vi "Do Request.vi"(7 "Processing In":refnum<class "Processing.lvclass">, 11 "ConfigHTTPController in":refnum<class "ConfigHTTPController.lvclass">) -> (0 "error out":errorcluster, 5 "Processing":refnum<class "Processing.lvclass">)   [LabVIEW 2023, in "Volatus.lvlib" / "ConfigHTTPController.lvclass"]
doc: "A controller's main job is to respond to a request by generating a response. The response value must be specified by calling Set Response.vi on the Processing class that's passed through the VI otherwise an error will be generated.\n\nThere are several helpers available for common response types:\nGenerating HTML content programmatically - Create Basic Response.vi\nStreaming a file from disk - Create File Response.vi\nRedirecting the user to another URL - Create Redirect Response.vi\n\nFile responses are streamed in chunks and do not load the entire file into memory at once to send in the response which allows serving large files more efficiently."
uses:
  ConfigHTTPController.lvclass
  lv-http-server/HTTP Server/Processing/Processing.lvclass
  lv-http-server/HTTP Server/Processing/Processing.lvclass/Processing.ctl
  lv-http-util/HTTP Utils/Request/Request.lvclass/Request.ctl
  lv-uri/URI/URI/URI.lvclass/URI.ctl
  ConfigInfoValue/ConfigInfoValue.lvclass
  ConfigHTTPController.lvclass/ConfigHTTPController.ctl
  MessageQ/MessageQ.lvclass/MessageQ.ctl
  lv-http-util/HTTP Utils/Request/Get Target URI.vi
  lv-uri/URI/URI/Path String.vi
  lv-http-util/HTTP Utils/File Response/File Response.lvclass
  MessageQ/MessageQ.lvclass
  lv-http-util/HTTP Utils/Response/Response.lvclass
  lv-http-util/HTTP Utils/Request/Request.lvclass
  lv-http-util/HTTP Utils/FormField/FormField.lvclass
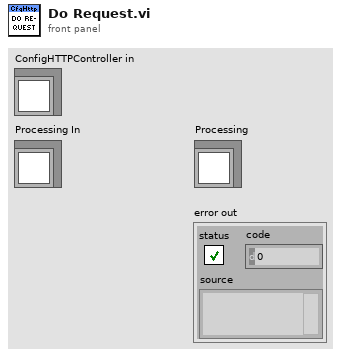
[diagram p1: front panel]
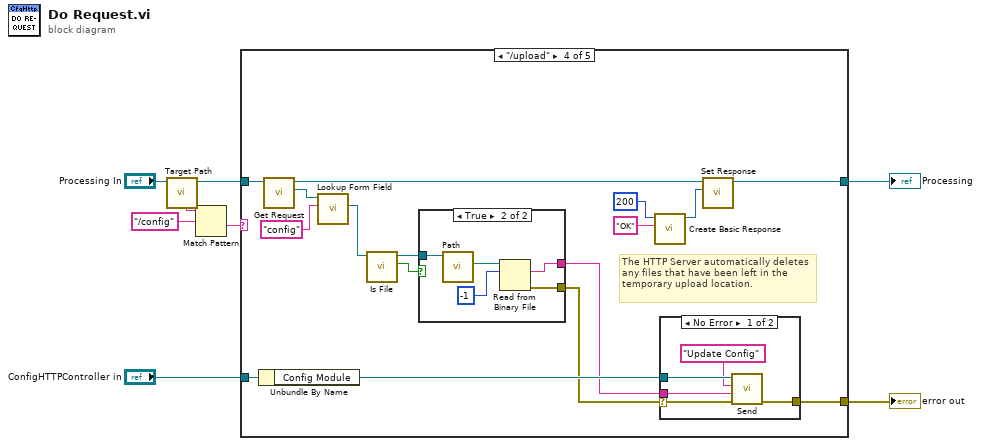
[diagram p0: block diagram]
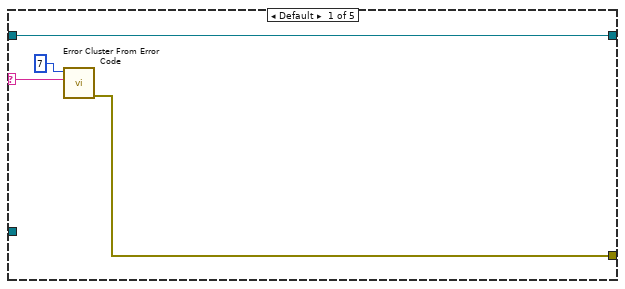
[diagram p2: hidden frame]
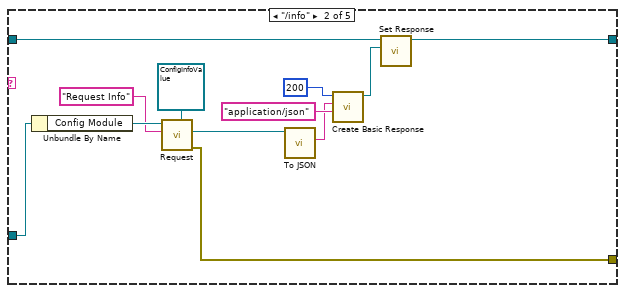
[diagram p3: hidden frame]
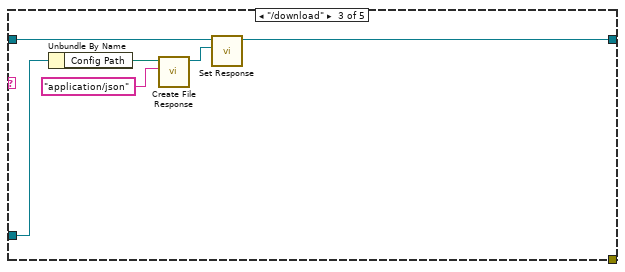
[diagram p4: hidden frame]
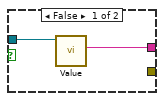
[diagram p6: hidden frame]
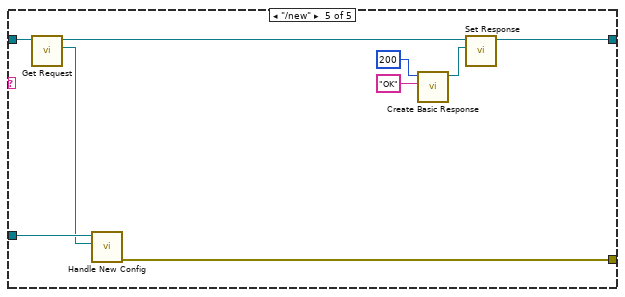
[diagram p7: hidden frame]
diagram:
  n1 = call "Target Path.vi"("Processing in"="Processing In") -> ("Processing out"=w3:refnum<class "Processing.lvclass">, "Target Path"=w7:string)  [unwired: 9 in]
  n2 = Match Pattern(string=w7, regular expression="/config") -> (after substring=w5:string)  [unwired: 1 in, 3 out]
  n3 = case shown="\"/upload\"" w5 {
    selector: w5 -> [w12 _ _ _ _]
    tunnel: [w10 w13 _ w41 w66] -> w4
    tunnel: w3 -> [w9 w16 w27 w46 w68]
    tunnel: "ConfigHTTPController in" -> [_ w24 w30 w43 w67]
    tunnel: [w9 w14 w25 w32 w60] -> w1
    frame Default {
      n4 = call <vilib>:"Error Cluster From Error Code.vi"("error message (\"\")"=w12, "error code (0)"=7) -> ("error out"=w10:errorcluster)  [unwired: 7 in]
    }
    frame "/info" {
      n5 = Unbundle By Name(w24) -> ("Config Module"=w23:refnum<class "MessageQ.lvclass">)
      n6 = call "Request.vi"("Response Type (None)"=refnum<class "ConfigInfoValue.lvclass"> refnum ("Volatus:ConfigInfoValue.lvclass"), "ID"="Request Info", "MessageQ in"=w23) -> ("error out"=w13:errorcluster, "Response"=w20:refnum<class "ConfigInfoValue.lvclass">)  [unwired: 6 in, 1 out]
      n7 = call "To JSON.vi"("ConfigInfoValue in"=w20) -> ("JSON string"=w17:string)  [unwired: 10 in]
      n8 = call "Create Basic Response.vi"("Content-Type (text/plain)"="application/json", "Payload"=w17, "Status Code"=u16 200) -> ("Response out"=w15:refnum<class "Response.lvclass">)  [unwired: 7 in, 1 out]
      n9 = call "Set Response.vi"("Response"=w15, "Processing in"=w16) -> ("Processing out"=w14:refnum<class "Processing.lvclass">)  [unwired: 9 in]
    }
    frame "/download" {
      n10 = Unbundle By Name(w30) -> ("Config Path"=w29:path)
      n11 = call "Create File Response.vi"("Content-Type (Auto)"="application/json", "Path"=w29) -> ("File Response out"=w26:refnum<class "File Response.lvclass">)  [unwired: 8 in, 1 out]
      n12 = call "Set Response.vi"("Response"=w26, "Processing in"=w27) -> ("Processing out"=w25:refnum<class "Processing.lvclass">)  [unwired: 9 in]
    }
    frame "/upload" {
      # "The HTTP Server automatically deletes any files that have been left in the temporary upload location."
      n13 = Unbundle By Name(w43) -> ("Config Module"=w42:refnum<class "MessageQ.lvclass">)
      n14 = call "Get Request.vi"("Processing in"=w46) -> ("Request"=w45:refnum<class "Request.lvclass">, "Processing out"=w44:refnum<class "Processing.lvclass">)  [unwired: 9 in]
      n15 = call "Lookup Form Field.vi"("Name"="config", "Request in"=w45) -> ("Field"=w38:refnum<class "FormField.lvclass">)  [unwired: 6 in, 3 out]
      n16 = call "Is File.vi"("FormField in"=w38) -> ("Is File?"=w37:bool, "FormField out"=w36:refnum<class "FormField.lvclass">)  [unwired: 8 in, 1 out]
      n17 = case shown="True" w37 {
        tunnel: [w54 w56] -> w39
        tunnel: w36 -> [w53 w59]
        tunnel: [_ w55] -> w35
        frame False {
          n18 = call "Value.vi"("FormField in"=w53) -> ("Value"=w54:string)  [unwired: 8 in, 2 out]
        }
        frame True {
          n19 = call "Path.vi"("FormField in"=w59) -> ("Path"=w58:path)  [unwired: 8 in, 2 out]
          n20 = Read from Binary File(10:-1 ("count (1)"), 11:w58) -> (0:w55:errorcluster, 2:w56:string)  [unwired: 4 in, 2 out]
        }
      }
      n21 = call "Create Basic Response.vi"("Payload"="OK", "Status Code"=u16 200) -> ("Response out"=w31:refnum<class "Response.lvclass">)  [unwired: 8 in, 1 out]
      n22 = case shown="No Error" w35 {
        selector: w35 -> [w47 w52]
        tunnel: w42 -> [w51 _]
        tunnel: [w49 w52] -> w41
        tunnel: w39 -> [w48 _]
        frame No Error {
          n23 = call "Send.vi"("error in (no error)"=w47, "Data"=w48, "ID"="Update Config", "MessageQ in"=w51) -> ("error out"=w49:errorcluster)  [unwired: 6 in, 1 out]
        }
        frame Error {
        }
      }
      n24 = call "Set Response.vi"("Response"=w31, "Processing in"=w44) -> ("Processing out"=w32:refnum<class "Processing.lvclass">)  [unwired: 9 in]
    }
    frame "/new" {
      n25 = call "Get Request.vi"("Processing in"=w68) -> ("Request"=w65:refnum<class "Request.lvclass">, "Processing out"=w61:refnum<class "Processing.lvclass">)  [unwired: 9 in]
      n26 = call "Handle New Config.vi"("Request"=w65, "ConfigHTTPController in"=w67) -> ("error out"=w66:errorcluster)  [unwired: 8 in, 1 out]
      n27 = call "Create Basic Response.vi"("Payload"="OK", "Status Code"=u16 200) -> ("Response out"=w62:refnum<class "Response.lvclass">)  [unwired: 8 in, 1 out]
      n28 = call "Set Response.vi"("Response"=w62, "Processing in"=w61) -> ("Processing out"=w60:refnum<class "Processing.lvclass">)  [unwired: 9 in]
    }
  }
  "error out" <- w4
  "Processing" <- w1
